vi "Clip common string ends.vi"(2 "Desired String Length":i32=35, 3 "String In":string[](array[string])) -> (1 "Clipped String":string[](array[string]))   [LabVIEW 2022 SP3]
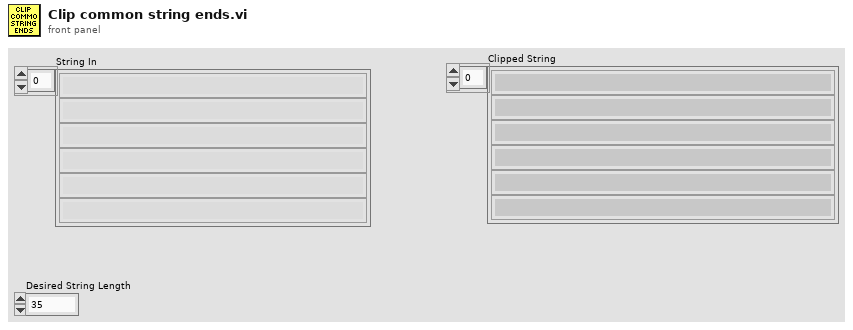
[diagram p1: front panel]
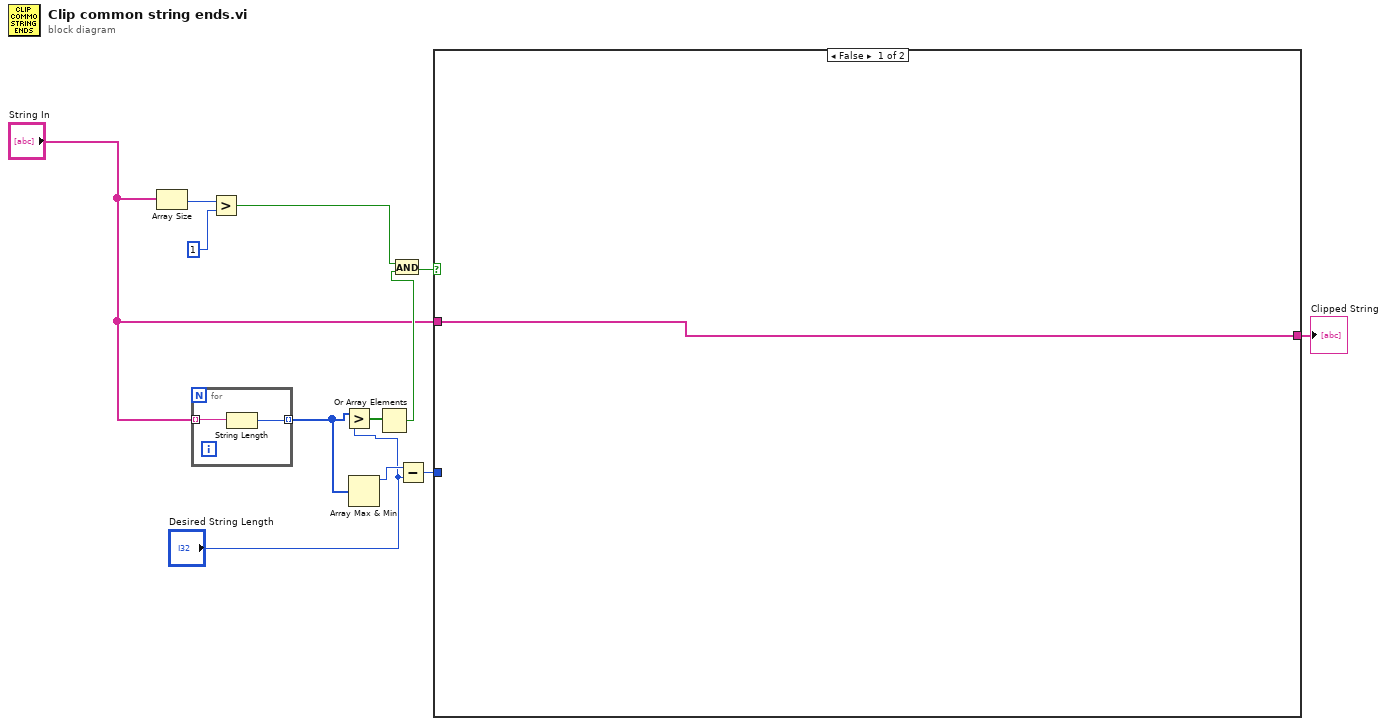
[diagram p0: block diagram]
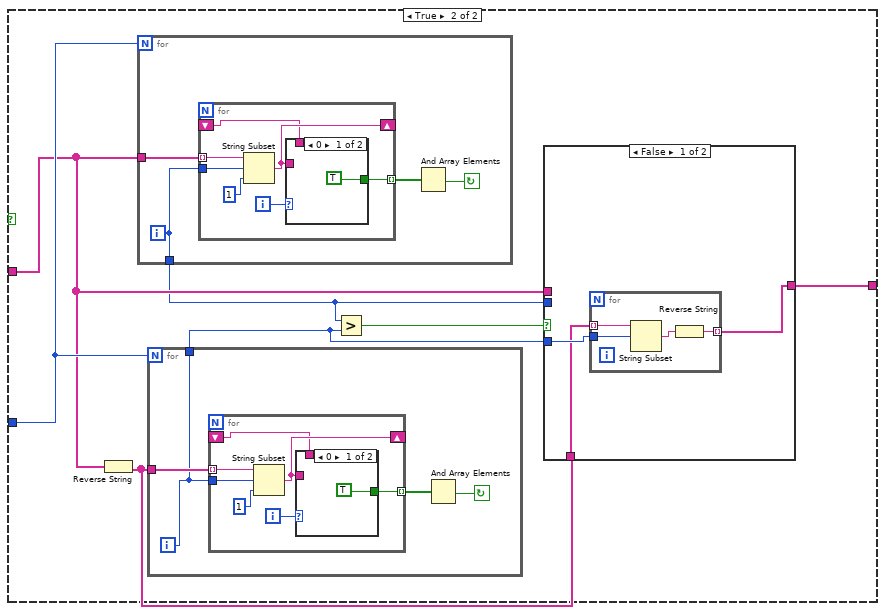
[diagram p2: hidden frame]
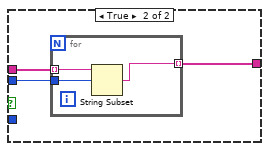
[diagram p3: hidden frame]
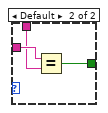
[diagram p4: hidden frame]
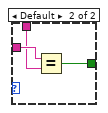
[diagram p5: hidden frame]
diagram:
  n1 = Array Size(array="String In") -> (size(s)=w11:i32)
  n2 = for {
    tunnel: "String In" -> [w14] mode=indexing
    tunnel: [w13] -> w6 mode=indexing
    n3 = String Length(string=w14) -> (length=w13:i32)
  }
  n4 = Greater?(x=w11, y=1) -> (0:w8:bool)
  n5 = Greater?(x=w6, y="Desired String Length") -> (0:w12:bool[])
  n6 = Array Max & Min(array=w6) -> (max value=w5:i32)  [unwired: 3 out]
  n7 = Or Array Elements(Boolean array=w12) -> (logical OR=w9:bool)
  n8 = And(x=w8, y=w9) -> (x .and. y?=w7:bool)
  n9 = Subtract(x=w5, y="Desired String Length") -> (x-y=w4:i32)
  n10 = case shown="False" w7 {
    tunnel: [w15 w20] -> w3
    tunnel: "String In" -> [w15 w21]
    tunnel: w4 -> [_ w22]
    frame False {
    }
    frame True {
      n11 = Reverse String(1:w21) -> (0:w16:string[])
      n12 = for {
        N: w22 -> [_]
        tunnel: w21 -> [w53]
        tunnel: [w51] -> w18
        i -> [w51]
        stop <- w52 continue-if-true
        n13 = for {
          tunnel: w53 -> [w61] mode=indexing
          shift-right: [w59] -> _
          shift-left: _ -> [w58]
          tunnel: [w56] -> w54 mode=indexing
          tunnel: w51 -> [w55]
          i -> [w60]
          n14 = String Subset(string=w61, offset (0)=w55, length (rest)=1 ("length (rest)")) -> (substring=w59:string)
          n15 = case shown="0" w60 {
            tunnel: w59 -> [_ w65]
            tunnel: w58 -> [_ w64]
            tunnel: [TRUE w63] -> w56
            frame 0 {
            }
            frame Default {
              n16 = Equal?(x=w65, y=w64) -> (x = y?=w63:bool)
            }
          }
        }
        n17 = And Array Elements(Boolean array=w54) -> (logical AND=w52:bool)
      }
      n18 = for {
        N: w22 -> [_]
        tunnel: w16 -> [w38]
        tunnel: [w36] -> w17
        i -> [w36]
        stop <- w37 continue-if-true
        n19 = for {
          tunnel: w38 -> [w46] mode=indexing
          shift-right: [w44] -> _
          shift-left: _ -> [w43]
          tunnel: [w41] -> w39 mode=indexing
          tunnel: w36 -> [w40]
          i -> [w45]
          n20 = String Subset(string=w46, offset (0)=w40, length (rest)=1 ("length (rest)")) -> (substring=w44:string)
          n21 = case shown="0" w45 {
            tunnel: w44 -> [_ w50]
            tunnel: w43 -> [_ w49]
            tunnel: [TRUE w48] -> w41
            frame 0 {
            }
            frame Default {
              n22 = Equal?(x=w50, y=w49) -> (x = y?=w48:bool)
            }
          }
        }
        n23 = And Array Elements(Boolean array=w39) -> (logical AND=w37:bool)
      }
      n24 = Greater?(x=w18, y=w17) -> (0:w19:bool)
      n25 = case shown="False" w19 {
        tunnel: w18 -> [_ w32]
        tunnel: w21 -> [_ w31]
        tunnel: [w23 w30] -> w20
        tunnel: w17 -> [w25 _]
        tunnel: w16 -> [w24 _]
        frame False {
          n26 = for {
            tunnel: w25 -> [w29]
            tunnel: w24 -> [w28] mode=indexing
            tunnel: [w26] -> w23 mode=indexing
            n27 = String Subset(string=w28, offset (0)=w29) -> (substring=w27:string)  [unwired: 1 in]
            n28 = Reverse String(1:w27) -> (0:w26:string)
          }
        }
        frame True {
          n29 = for {
            tunnel: w32 -> [w35]
            tunnel: w31 -> [w34] mode=indexing
            tunnel: [w33] -> w30 mode=indexing
            n30 = String Subset(string=w34, offset (0)=w35) -> (substring=w33:string)  [unwired: 1 in]
          }
        }
      }
    }
  }
  "Clipped String" <- w3
